vi "Delete_From_Array.vi"(0 "Choose delete from array":T2, 1 "Length":i32, 2 "Index Delete":i32, 3 "Delete from Array 1D":i8[](array[numeric])=[0, 1, 2, 3, 4], 4 "Indexs DFA":T1={"Rows"=-1, "Columns"=-1} {"Columns" min=-1; "Rows" min=-1}, 5 "Delete from Array 2D":i8[][](array[numeric])=[[-5, -1, 3], [-4, 0, 4], [-3, 1, 5], [-2, 2, 6]]) -> (15 "New Array 1D":i8[](array[numeric]), 16 "Deleted Portion 1D":i8[](array[numeric]), 17 "New Array 2D":i8[][](array[numeric]), 18 "Deleted Portion 2D":i8[][](array[numeric]))   [LabVIEW 2018]
uses:
  Controls/1D_2D.ctl
  Controls/Rows_Columns.ctl
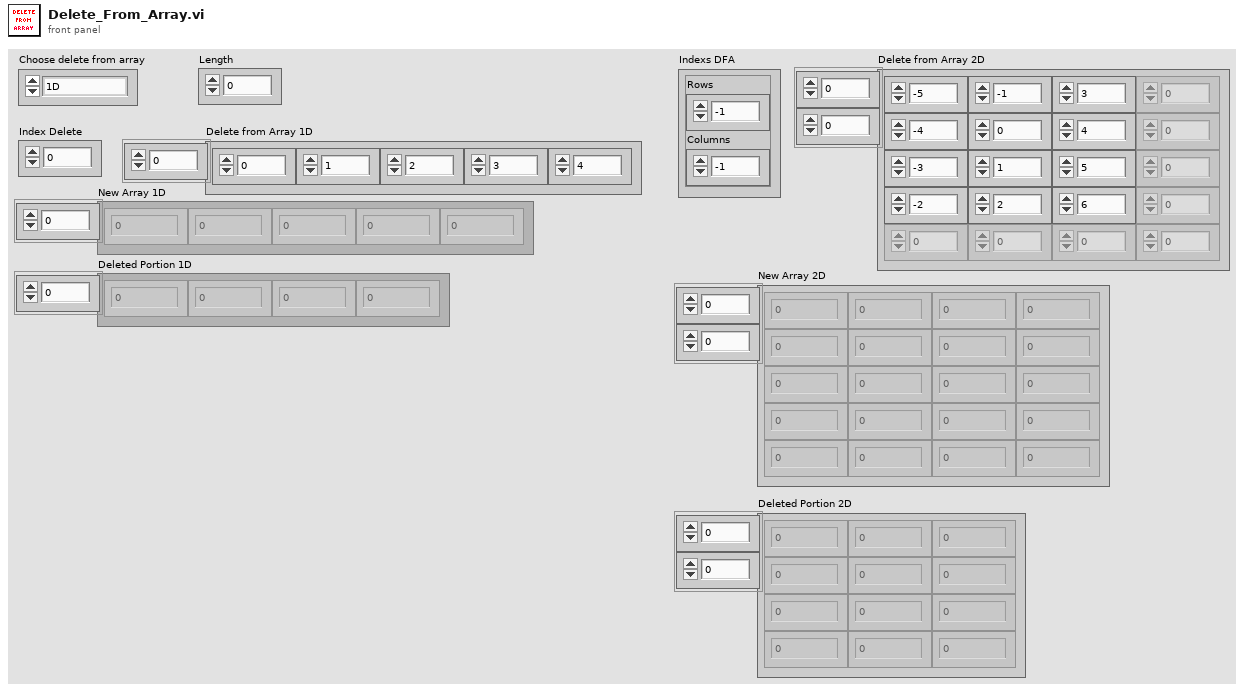
[diagram p1: front panel]
types:
  T1 = typedef "Rows_Columns.ctl" = cluster{"Rows":i32, "Columns":i32}
  T2 = typedef "1D_2D.ctl" = enum16{"1D", "2D"}
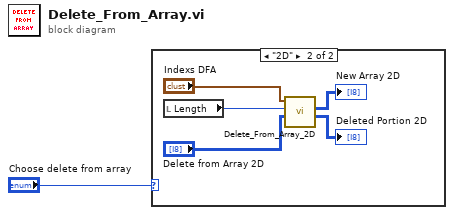
[diagram p0: block diagram]
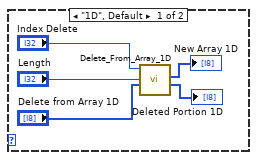
[diagram p2: hidden frame]
diagram:
  n1 = case shown="\"2D\"" "Choose delete from array" {
    frame "1D", Default {
      n2 = call "Delete_From_Array_1D.vi"("Delete from Array 1D"="Delete from Array 1D", "Length"="Length", "Index Delete"="Index Delete") -> ("Deleted Portion 1D"=→"Deleted Portion 1D":i8[], "New Array 1D"=→"New Array 1D":i8[])  [unwired: 7 in]
    }
    frame "2D" {
      n3 = local read "Length"() -> (w10:i32)
      n4 = call "Delete_From_Array_2D.vi"("Delete from Array 2D"="Delete from Array 2D", "length"=w10, "Indexs DFA"="Indexs DFA") -> ("Deleted Portion 2D"=→"Deleted Portion 2D":i8[][], "New Array 2D"=→"New Array 2D":i8[][])  [unwired: 7 in]
    }
  }
